vi "2D Commands.vi"(0 "2D wavename":string="datatest.000016", 5 "X wavename":string="xx", 7 "Y wavename":string="yy", 9 "X,Y,Z Labels":string[](array[string])=["current (nA)", "field (oe)", "dV/dI (Ohm)"], 13 "input string":string="Display;AppendImage '#wave2D#'\nModifyGraph width=216,height={Aspect,1}\nLabel bottom \"#labelX#\"\nLabel left \"#labelY#\"\nModifyImage '#wave2D#' ctab= {*,*,Rainbow,1}\nModifyGraph mirror=1") -> (4 "result string":string="Display;AppendImage 'datatest.000016'\nModifyGraph width=216,height={Aspect,1}\nLabel bottom \"current (nA)\"\nLabel left \"field (oe)\"\nModifyImage 'datatest.000016' ctab= {*,*,Rainbow,1}\n")   [LabVIEW 2016, in "LV to ITX.lvclass"]
uses:
  LV to ITX.lvclass
panel:
  # "Display;AppendImage '#wave2D#'\nModifyGraph width=216,height={Aspect,1}\nLabel bottom \"#labelX#\"\nLabel left \"#labelY#\"\nModifyImage '#wave2D#' ctab= {*,*,BlueHot,1}"
  # "Display;AppendImage '#wave2D#'\nModifyGraph width=216,height={Aspect,1}\nLabel bottom \"#labelX#\"\nLabel left \"#labelY#\"\nModifyImage '#wave2D#' ctab= {120,300,BlueHot,1}"
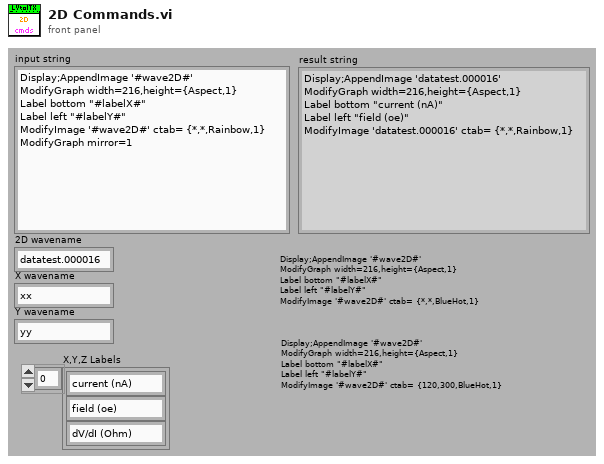
[diagram p1: front panel]
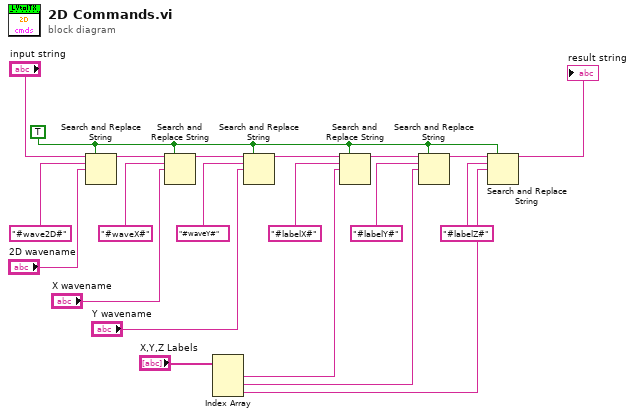
[diagram p0: block diagram]
diagram:
  w8 = TRUE ("replace all? (F)")
  n1 = Search and Replace String(replace all?=w8, input string="input string", search string="#wave2D#", replace string="2D wavename") -> (result string=w14:string)  [unwired: 1 in, 6 out]
  n2 = Search and Replace String(replace all?=w8, input string=w14, search string="#waveX#", replace string="X wavename") -> (result string=w16:string)  [unwired: 1 in, 6 out]
  n3 = Index Array(array="X,Y,Z Labels") -> (element #1=w3:string, element #2=w5:string, element #3=w4:string)  [unwired: 3 in]
  n4 = Search and Replace String(replace all?=w8, input string=w16, search string="#waveY#", replace string="Y wavename") -> (result string=w9:string)  [unwired: 1 in, 6 out]
  n5 = Search and Replace String(replace all?=w8, input string=w9, search string="#labelX#", replace string=w3) -> (result string=w12:string)  [unwired: 1 in, 6 out]
  n6 = Search and Replace String(replace all?=w8, input string=w12, search string="#labelY#", replace string=w5) -> (result string=w6:string)  [unwired: 1 in, 6 out]
  n7 = Search and Replace String(replace all?=w8, input string=w6, search string="#labelZ#", replace string=w4) -> (result string=→"result string":string)  [unwired: 1 in, 6 out]
